vi "Delete User.vi"(10 "User Type":string, 11 "Path":path=path "E:/labview code/project user login/test1.txt") -> ()   [LabVIEW 2015]
panel:
  in  "SELECT USER NAME":u16(ring) items=["asd"]
  in  "delete":bool
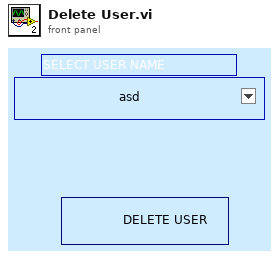
[diagram p1: front panel]
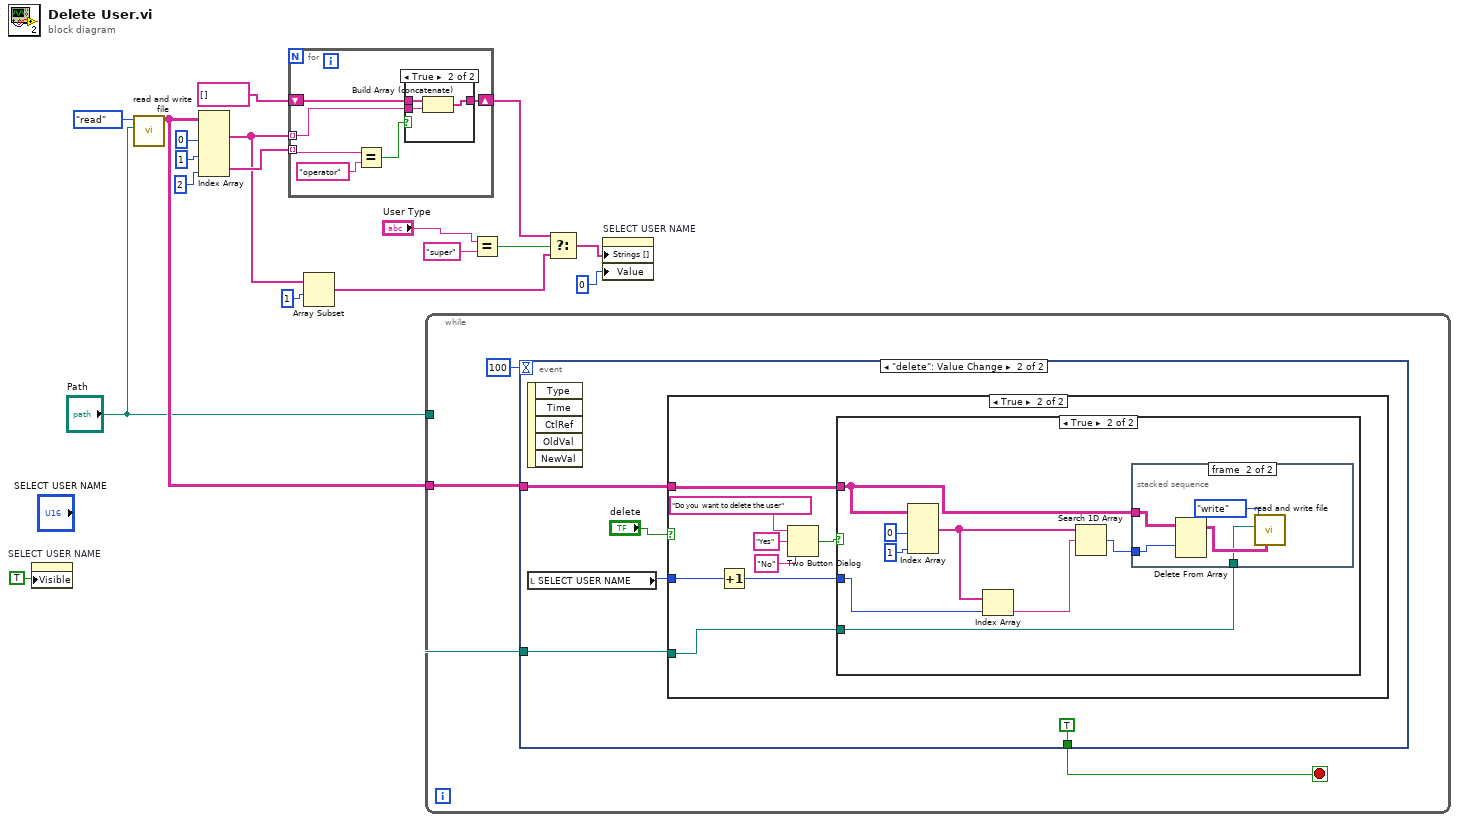
[diagram p0: block diagram]
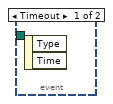
[diagram p3: hidden frame]
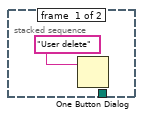
[diagram p6: hidden frame]
diagram:
  n1 = property on="SELECT USER NAME" class="Ring (strict)"("Visible"=TRUE) -> ()  [unwired: 2 in, 2 out]
  n2 = call "read and write file.vi"("Path"="Path", "Enum"=enum16{"write", "read"}."read") -> ("output data"=w11:string[][])  [unwired: 9 in]
  n3 = Index Array(array=w11, index (col) #1=0 ("index (row)"), index (col) #2=1 ("index (row)"), index (col) #3=2 ("index (col)")) -> (element #1=w6:string[], element #3=w7:string[])  [unwired: 3 in, 1 out]
  n4 = for {
    tunnel: w7 -> [w24] mode=indexing
    tunnel: w6 -> [w21] mode=indexing
    shift-right: [w22] -> w3
    shift-left: string[] [] ("subarray") -> [w20]
    n5 = Equal?(x=w24, y="operator") -> (x = y?=w19:bool)
    n6 = case shown="True" w19 {
      tunnel: [w25 w28] -> w22
      tunnel: w21 -> [_ w27]
      tunnel: w20 -> [w25 w26]
      frame False {
      }
      frame True {
        n7 = Build Array (concatenate)(w26, w27) -> (w28:string[])
      }
    }
  }
  n8 = Array Subset(array=w6, index=1) -> (w2:string[])  [unwired: 1 in]
  n9 = while {
    tunnel: "Path" -> [w31]
    tunnel: w11 -> [w30]
    stop <- w32 stop-if-true
    n10 = event shown="[1] \"delete\": Value Change" {
      selector: _ -> [_ _]
      dyn-events: _ -> [_ _]
      timeout: 100 -> [_ _]
      tunnel: [_ TRUE ("Exit 2")] -> w32
      tunnel: w30 -> [_ w35]
      tunnel: w31 -> [_ w34]
      event Timeout {
        n11 = event-data() -> ()  [unwired: 1 in, 2 out]
      }
      event "delete": Value Change {
        n12 = event-data() -> ()  [unwired: 1 in, 5 out]
        n13 = local read "SELECT USER NAME"() -> (w37:u16)
        n14 = case shown="True" "delete" {
          tunnel: w37 -> [_ w45]
          tunnel: w35 -> [_ w40]
          tunnel: w34 -> [_ w38]
          frame False {
          }
          frame True {
            n15 = Increment(x=w45) -> (x+1=w39:u16)
            n16 = Two Button Dialog(message="Do you  want to delete the user", 1:"No" ("F button name (\"Cancel\")"), 2:"Yes" ("T button name (\"OK\")")) -> (T button?=w44:bool)
            n17 = case shown="True" w44 {
              tunnel: w39 -> [_ w48]
              tunnel: w40 -> [_ w47]
              tunnel: w38 -> [_ w46]
              frame False {
              }
              frame True {
                n18 = Index Array(array=w47, index (col) #1=0 ("index (row)"), index (col) #2=1 ("index (row)")) -> (element #1=w50:string[])  [unwired: 2 in, 1 out]
                n19 = Index Array(array=w50, index=w48) -> (element=w49:string)
                n20 = Search 1D Array(1D array=w50, element=w49) -> (index of element=w51:i32)  [unwired: 1 in]
                n21 = stacked-sequence {
                  tunnel: w51 -> [_ w59]
                  tunnel: w47 -> [_ w58]
                  tunnel: w46 -> [_ w55]
                  frame #0 {
                    n22 = One Button Dialog(message="User delete") -> ()  [unwired: 1 in, 1 out]
                  }
                  frame #1 {
                    n23 = Delete From Array(array=w58, index (row)=w59) -> (array with subset deleted=w57:string[][])  [unwired: 2 in, 1 out]
                    n24 = call "read and write file.vi"("data to write"=w57, "Path"=w55, "Enum"=enum16{"write", "read"}."write") -> ()  [unwired: 8 in, 1 out]
                  }
                }
              }
            }
          }
        }
      }
    }
  }
  n25 = Equal?(x="User Type", y="super") -> (x = y?=w4:bool)
  n26 = Select(t=w3, s=w4, f=w2) -> (s? t:f=w1:string[])
  n27 = property on="SELECT USER NAME" class="Ring (strict)"("Strings []"=w1, "Value"=u16 0 ("index")) -> ()  [unwired: 2 in, 2 out]
